vi "4.2.-Histograma Sin Case Structure.vi"() -> ()   [LabVIEW 2020]
panel:
  out "Azul":dbl
  out "Verde":dbl
  out "Rojo":dbl
  out "Waveform Graph":dbl[][](graph)
  out "Sample taken":picture
  in  "Sample Size":dbl(knob) scale=0.0..100.0
  out "Image":picture
  in  "Path":path
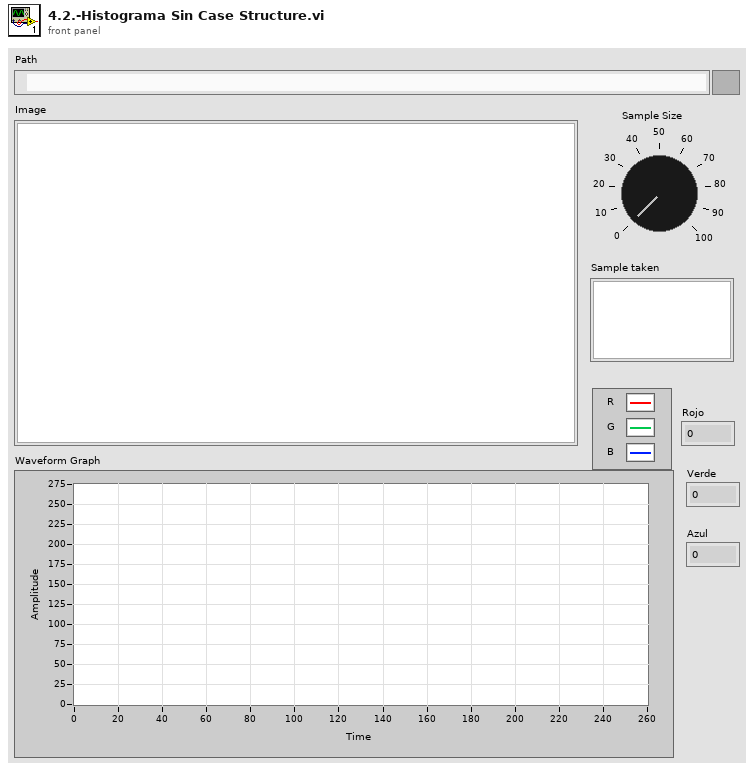
[diagram p1: front panel]
types:
  T1 = typedef "imagedata.ctl" = cluster{"image type":i32, "image depth":i32, "image":u8[], "mask":u8[], "colors":u32[], "Rectangle":cluster{"left":i16, "top":i16, "right":i16, "bottom":i16}}
  T2 = typedef "LVMouseTypeDef.ctl" = cluster{"Mouse Position":cluster{"X":i32, "Y":i32}, "Mouse Modifiers":cluster{"Button Down":bool, "Shift Mod":bool, "Menu Mod":bool, "Option Mod":bool}}
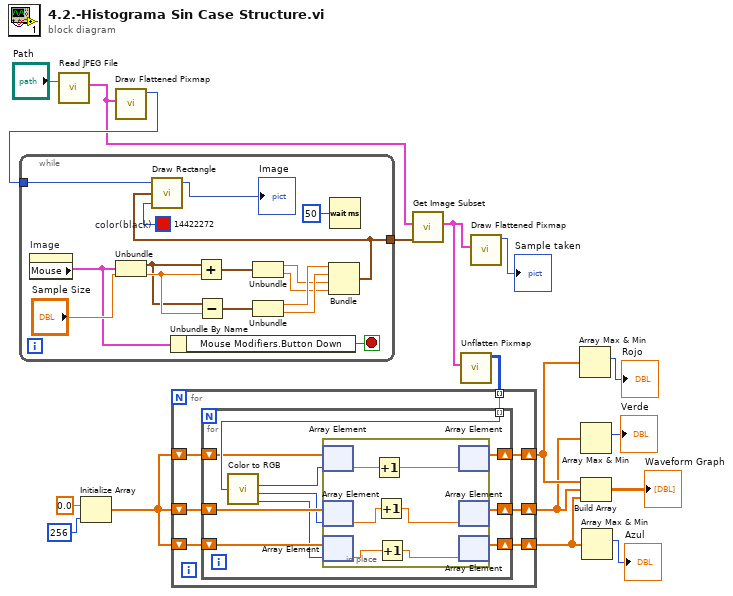
[diagram p0: block diagram]
diagram:
  n1 = call <vilib>:"Read JPEG File.vi"("path to JPEG file"="Path") -> ("image data"=w14:T1)  [unwired: 8 in, 2 out]
  n2 = Initialize Array "Initialize Array"(0.0 ("element"), 256 ("dimension size")) -> (w8:dbl[])
  n3 = call <vilib>:"Draw Flattened Pixmap.vi"("image data"=w14) -> ("new picture"=w16:picture)  [unwired: 8 in]
  n4 = while {
    tunnel: w16 -> [w31]
    tunnel: [w20] -> w15
    stop <- w18 stop-if-true
    w21 = u32 14422272  # color(black)
    n5 = property on="Image" class="Pict"() -> ("Mouse"=w19:T2)  [unwired: 2 in, 2 out]
    n6 = Unbundle "Unbundle"(w19) -> ("Mouse Position"=w26:cluster{"X":i32, "Y":i32})  [unwired: 1 out]
    n7 = Unbundle By Name "Unbundle By Name"(w19) -> ("Mouse Modifiers.Button Down"=w18:bool)
    n8 = Add(x=w26, y="Sample Size") -> (x+y=w29:cluster{"X":dbl, "Y":dbl})
    n9 = Subtract(x=w26, y="Sample Size") -> (x-y=w28:cluster{"X":dbl, "Y":dbl})
    n10 = Unbundle "Unbundle"(w29) -> ("X"=w23:dbl, "Y"=w22:dbl)
    n11 = Unbundle(w28) -> ("X"=w25:dbl, "Y"=w24:dbl)
    n12 = Bundle "Bundle"("X"=w25, "Y"=w24, "X"=w23, "Y"=w22) -> (w20:cluster{"X":dbl, "Y":dbl, "X":dbl, "Y":dbl})  [unwired: 1 in]
    n13 = call <vilib>:"Draw Rectangle.vi"("picture"=w31, "rect"=w20, "color(black)"=w21) -> ("new picture"=→"Image":picture)  [unwired: 6 in]
    n14 = Wait (ms)(milliseconds to wait=u32 50) -> ()  [unwired: 1 out]
  }
  n15 = call <vilib>:"Get Image Subset.vi"("subset rect"=w15, "image data"=w14) -> ("image subset"=w12:T1)  [unwired: 4 in, 1 out]
  n16 = call <vilib>:"Unflatten Pixmap.vi"("image data"=w12) -> ("24-bit pixmap"=w11:u32[][])  [unwired: 4 in, 6 out]
  n17 = for {
    tunnel: w11 -> [w39] mode=indexing
    shift-right: [w35] -> w6
    shift-left: w8 -> [w38]
    shift-right: [w33] -> w3
    shift-left: w8 -> [w37]
    shift-right: [w34] -> w1
    shift-left: w8 -> [w36]
    n18 = for {
      tunnel: w39 -> [w49] mode=indexing
      shift-right: [w46] -> w35
      shift-left: w38 -> [w48]
      shift-right: [w40] -> w33
      shift-left: w37 -> [w45]
      shift-right: [w41] -> w34
      shift-left: w36 -> [w43]
      n19 = call <vilib>:"Color to RGB.vi"("Color"=w49) -> ("R"=w47:u8, "G"=w44:u8, "B"=w42:u8)  [unwired: 1 out]
      n20 = in-place "In Place Element Structure" {
        n21 = in-place-array #1(w48, w47) -> (w55:dbl)
        n22 = in-place-array #2(w45, w44) -> (w53:dbl)
        n23 = in-place-array #3(w43, w42) -> (w51:dbl)
        n24 = Increment(x=w55) -> (x+1=w54:dbl)
        n25 = Increment(x=w53) -> (x+1=w52:dbl)
        n26 = Increment(x=w51) -> (x+1=w50:dbl)
        n27 = in-place-array #1(w54) -> (w46:dbl[])  [unwired: 1 out]
        n28 = in-place-array #2(w52) -> (w40:dbl[])  [unwired: 1 out]
        n29 = in-place-array #3(w50) -> (w41:dbl[])  [unwired: 1 out]
      }
    }
  }
  n30 = call <vilib>:"Draw Flattened Pixmap.vi"("image data"=w12) -> ("new picture"=→"Sample taken":picture)  [unwired: 8 in]
  n31 = Array Max & Min(array=w6) -> (max index (indices)=→"Rojo":i32)  [unwired: 3 out]
  n32 = Array Max & Min(array=w3) -> (max index (indices)=→"Verde":i32)  [unwired: 3 out]
  n33 = Build Array "Build Array"(w6, w3, w1) -> (→"Waveform Graph":dbl[][])
  n34 = Array Max & Min(array=w1) -> (max index (indices)=→"Azul":i32)  [unwired: 3 out]
